vi "环境参数table定义.vi"(10 "table 输入":string, 11 "data":cluster{"时间标识":timestamp, "监测值":sgl, "单位":u16} {"单位" items=["ug/L", "mg/L", "ppm", "mg/m3", "cm", "ppb", "ug/m3", "%", "nmol/mol", "umol/mol", "MPN/L", "MPN/100ml", "ng/m3", "NTU", "无量纲", "ms/cm", "us/cm", "℃", "V", "m3/s", "m3", "m", "m/s"]}) -> (1 "table 输出":string, 2 "columns":string[](array[string]), 3 "data输出":T1)   [LabVIEW 2016, in "database.lvlib"]
uses:
  database.lvlib
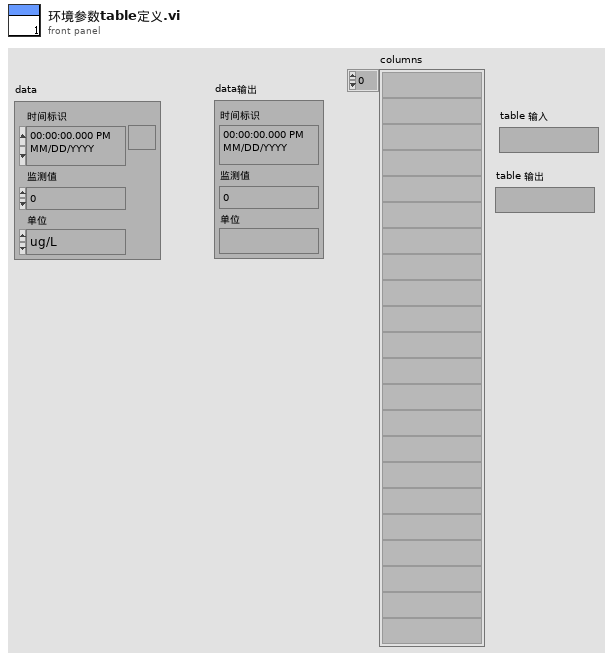
[diagram p1: front panel]
types:
  T1 = cluster{"时间标识":timestamp, "监测值":sgl, "单位":string}
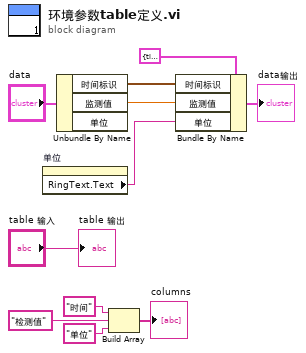
[diagram p0: block diagram]
diagram:
  n1 = property on="单位" class="Ring (严格)"() -> ("RingText.Text"=w6:string)  [unwired: 2 in, 2 out]
  n2 = Unbundle By Name("data") -> ("时间标识"=w8:timestamp, "监测值"=w7:sgl)  [unwired: 1 out]
  n3 = Build Array("时间", "检测值", "单位") -> (→"columns":string[])
  n4 = Bundle By Name(cluster=T1 {"时间标识"=timestamp(0 s since 1904-01-01), "监测值"=0.0, "单位"=""} ("data输出"), "时间标识"=w8, "监测值"=w7, "单位"=w6) -> (→"data输出":T1)
  "table 输出" <- "table 输入"
